vi "pmu_Check GPS Status.vi"(0 "GPS information":T2[](array[typedef]), 2 "reset? (F)":bool, 5 "data in":T1, 9 "system info in":refnum<class "PMU System Info.lvclass">, 11 "error in (no error)":errorcluster) -> (4 "GPS first locking?":bool, 8 "unlocked first index":i32, 10 "system info out":refnum<class "PMU System Info.lvclass">, 15 "error out":errorcluster)   [LabVIEW 2012, in "NI_EP_PMU.lvlib"]
doc: "Outputs time quality flag bits, according to IEEE Std C37.118."
uses:
  <vilib>/addons/Electrical Power/PMU/NI_EP_PMU.lvlib
  <vilib>/addons/Electrical Power/PMU/Common/Classes/PMU System Info/PMU System Info.lvclass
  <vilib>/addons/Electrical Power/PMU/Common/Controls/pmu_GPS Info.ctl
  <vilib>/addons/Electrical Power/PMU/Common/Controls/pmu_Phasor Measurement Data.ctl
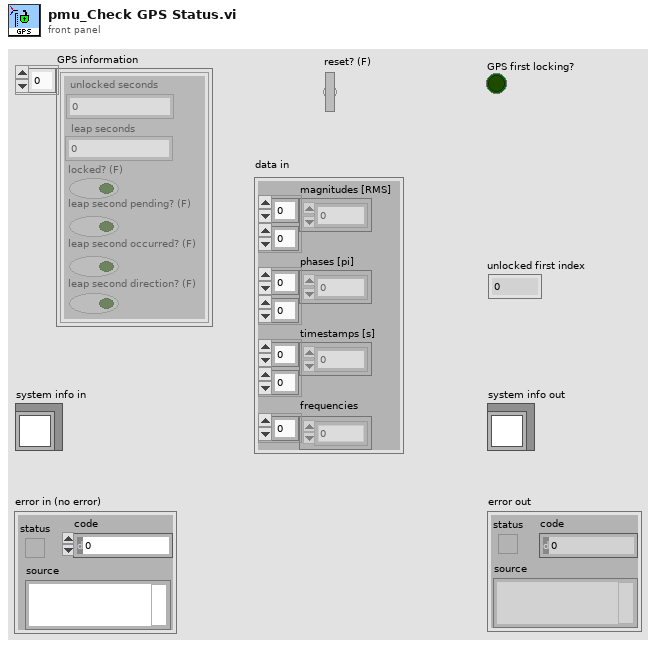
[diagram p1: front panel]
types:
  T1 = typedef "NI_EP_PMU.lvlib/pmu_Phasor Measurement Data.ctl" = cluster{"magnitudes [RMS]":dbl[][], "phases [pi]":dbl[][], "timestamps [s]":dbl[][], "frequencies":dbl[]}
  T2 = typedef "NI_EP_PMU.lvlib/pmu_GPS Info.ctl" = cluster{"unlocked seconds":u32, "leap seconds":i8, "locked? (F)":bool, "leap second pending? (F)":bool, "leap second occurred? (F)":bool, "leap second direction? (F)":bool}
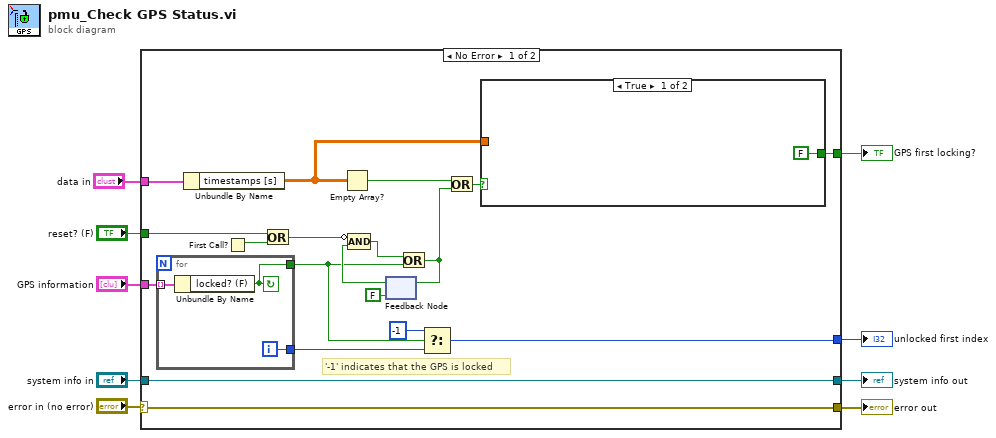
[diagram p0: block diagram]
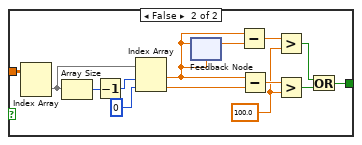
[diagram p2: hidden frame]
diagram:
  n1 = case shown="No Error" "error in (no error)" {
    selector: "error in (no error)" -> [w27 w47]
    tunnel: "GPS information" -> [w16 _]
    tunnel: "system info in" -> [w28 _]
    tunnel: [w27 w47] -> w9
    tunnel: [w28 _] -> w8
    tunnel: "reset? (F)" -> [w22 _]
    tunnel: [w18 _] -> w3
    tunnel: "data in" -> [w15 _]
    tunnel: [w10 _] -> w1
    frame No Error {
      # "'-1' indicates that the GPS is locked"
      n2 = for {
        tunnel: w16 -> [w46] mode=indexing
        tunnel: [w45] -> w20
        tunnel: [w44] -> w17
        i -> [w44]
        stop <- w45 continue-if-true
        n3 = Unbundle By Name(w46) -> ("locked? (F)"=w45:bool)
      }
      n4 = Unbundle By Name(w15) -> ("timestamps [s]"=w11:dbl[][])
      n5 = First Call?() -> (First Call?: T/F=w23:bool)
      n6 = Or(x=w22, y=w23) -> (x .or. y?=w21:bool)
      n7 = Empty Array?(array=w11) -> (empty?=w13:bool)
      n8 = feedback #1(FALSE) -> (w25:bool)
      n9 = Compound Arithmetic op=AND(invert w21, w25) -> (w24:bool)
      n10 = Or(x=w24, y=w20) -> (x .or. y?=w12:bool)
      n11 = feedback-in #1(w12) -> ()
      n12 = Select(t=-1, s=w20, f=w17) -> (s? t:f=w18:i32)
      n13 = Or(x=w13, y=w12) -> (x .or. y?=w14:bool)
      n14 = case shown="True" w14 {
        tunnel: [FALSE w34] -> w10
        tunnel: w11 -> [_ w30]
        frame True {
        }
        frame False {
          w35 = 100.0 ("y")
          n15 = Index Array(array=w30) -> (element=w31:dbl[])  [unwired: 2 in]
          n16 = Array Size(array=w31) -> (size(s)=w43:i32)
          n17 = Decrement(x=w43) -> (x-1=w42:i32)
          n18 = Index Array(array=w31, index #1=w42, index #2=0 ("index")) -> (element #1=w37:dbl, element #2=w40:dbl)
          n19 = feedback #2(w37) -> (w38:dbl)
          n20 = feedback-in #2(w37) -> ()
          n21 = Subtract(x=w37, y=w38) -> (x-y=w36:dbl)
          n22 = Subtract(x=w37, y=w40) -> (x-y=w39:dbl)
          n23 = Greater?(x=w36, y=w35) -> (0:w33:bool)
          n24 = Greater?(x=w39, y=w35) -> (0:w32:bool)
          n25 = Or(x=w33, y=w32) -> (x .or. y?=w34:bool)
        }
      }
    }
    frame Error {
    }
  }
  "error out" <- w9
  "system info out" <- w8
  "unlocked first index" <- w3
  "GPS first locking?" <- w1
